vi "2P_AdapUprite_Linlin.vi"() -> ()   [LabVIEW 2015] (continued)
                                n912 = disable-structure shown="Disabled" {
                                frame Disabled {
                                n913 = call "stoperaseCI.vi"() -> ()  [unwired: 12 in]
                                n914 = call "stoperaseDO_img.vi"() -> ()  [unwired: 12 in]
                                n915 = call "stoperaseAO_img.vi"() -> ()  [unwired: 12 in]
                                n916 = call "stoperaseAI_img.vi"() -> ()  [unwired: 12 in]
                                }
                                frame Enabled {
                                }
                                }
                                }
                                frame #1 {
                                n917 = disable-structure shown="Disabled" {
                                frame Disabled {
                                n918 = local read "Acquisition time"() -> (w3439:i32)
                                n919 = call "collect_allLT_img.vi"() -> ("counts"=w3441:i32)  [unwired: 1 out]
                                n920 = local read "counts"() -> (w3442:i32)
                                n921 = Add(x=w3442, y=w3441) -> (x+y=w3440:i32)
                                "counts" <- w3440
                                n922 = Divide(x=w3440, y=w3439) -> (x/y=w3438:dbl)
                                n923 = Multiply(x=1000.0, y=w3438) -> (x*y=w3437:dbl)
                                n924 = local write "Avg Counts/s"(w3437) -> ()
                                }
                                frame Enabled {
                                }
                                }
                                }
                                frame #2 {
                                w3445 = u16 0 items=["Stream to disk", "Post process", "real time process"] ("Ring")
                                n925 = local read "T3R Data processing"() -> (w3444:u16)
                                n926 = local read "save\ndata"() -> (w3447:bool)
                                n927 = Equal?(x=w3444, y=w3445) -> (x = y?=w3443:bool)
                                n928 = Not(x=w3443) -> (.not. x?=w3448:bool)
                                n929 = And(x=w3447, y=w3448) -> (x .and. y?=w3446:bool)
                                n930 = case shown="True" w3446 {
                                tunnel: w3449 -> [_ w3451]
                                frame False {
                                }
                                frame True {
                                n931 = local read "filename prefix"() -> (w3452:string)
                                n932 = local read "data dir"() -> (w3457:path)
                                n933 = call "2pparameters.vi"("command"="get") -> ("params out"=w3472:T12)  [unwired: 1 in]
                                n934 = call "generatedatafilename.vi"("timestamp"=w3451, "filename prefix in"=w3452) -> ("full-filename"=w3450:string)
                                n935 = Unbundle By Name(w3472) -> ("srate"=w3470:sgl, "sAOxy"=w3469:i32, "Xpixels Img"=w3467:i32, "Ypixels Img"=w3465:i32)
                                n936 = Concatenate Strings(w3450, ".lvpt3img" ("string")) -> (w3455:string)
                                n937 = Build Path(base path=w3457, name or relative path=w3455) -> (appended path=w3454:path)
                                n938 = To Unsigned Long Integer(number=w3470) -> (unsigned 32bit integer=w3471:u32)
                                n939 = To Unsigned Long Integer(number=w3469) -> (unsigned 32bit integer=w3468:u32)
                                n940 = To Unsigned Long Integer(number=w3467) -> (unsigned 32bit integer=w3466:u32)
                                n941 = To Unsigned Long Integer(number=w3465) -> (unsigned 32bit integer=w3464:u32)
                                n942 = call "PH-temp-raw.vi"("command"="get") -> ("array out"=w3463:u32[])  [unwired: 1 in]
                                n943 = Build Array (concatenate)(w3471, w3468, w3466, w3464, w3463) -> (w3462:u32[])
                                n944 = Open/Create/Replace File(file path (use dialog)=w3454, operation (0:open)=T9."replace or create") -> (refnum out=w3461:refnum<file>, error out=w3460:errorcluster)  [unwired: 4 in, 1 out]
                                n945 = Write to Binary File(file (use dialog)=w3461, data=w3462, error in=w3460, 5:FALSE ("prepend array or string size? (T)")) -> (refnum out=w3458:refnum<file>, error out=w3459:errorcluster)  [unwired: 2 in, 1 out]
                                n946 = Close File(refnum=w3458, error in=w3459) -> ()  [unwired: 2 out]
                                }
                                }
                                n947 = call "stoperaseLT_img.vi"() -> ()  [unwired: 1 in]
                                }
                                frame #3 {
                                w3478 = u16 1 items=["Stream to disk", "Post process", "real time process"] ("Ring")
                                n948 = local read "T3R Data processing"() -> (w3477:u16)
                                n949 = Equal?(x=w3477, y=w3478) -> (x = y?=w3476:bool)
                                n950 = case shown="True" w3476 {
                                frame False {
                                }
                                frame True {
                                # "intensity"
                                # "lifetime"
                                # "intensity"
                                n951 = property on="img_CH1" class="IntGraph (strict)"() -> ("Value"=w3491:sgl[][])  [unwired: 2 in, 2 out]
                                n952 = Array Max & Min(array=w3491) -> (max value=w3492:sgl)  [unwired: 3 out]
                                n953 = local read "lineshift"() -> (w3479:i32)
                                n954 = local read "min phot"() -> (w3493:u32)
                                n955 = To Unsigned Long Integer(number=w3492) -> (unsigned 32bit integer=w3495:u32)
                                n956 = local read "counts"() -> (w3481:i32)
                                n957 = call "wrapcutlifetime.vi"("lineshift"=w3479) -> ("pt3img"=w3490:u16[][], "lifetimes"=w3488:sgl[][], "okay"=w3483:bool, "# of frames"=w3480:i32)
                                "frames recorded" <- w3480
                                n958 = Greater?(x=w3493, y=w3495) -> (0:w3494:bool)
                                n959 = Quotient & Remainder(x=w3481, y=w3480) -> (floor(x/y)=w3482:i32)  [unwired: 1 out]
                                n960 = Transpose 2D Array(2D array=w3490) -> (transposed array=w3484:u16[][])
                                n961 = Transpose 2D Array(2D array=w3488) -> (transposed array=w3489:sgl[][])
                                n962 = And(x=w3494, y=w3483) -> (x .and. y?=w3496:bool)
                                n963 = local write "img_CH2"(w3489) -> ()
                                n964 = local write "photons/frame"(w3482) -> ()
                                n965 = Array Max & Min(array=w3484) -> (max value=w3485:u16)  [unwired: 3 out]
                                n966 = To Single Precision Float(number=w3484) -> (single precision float=w3487:sgl[][])
                                n967 = case shown="True" w3496 {
                                tunnel: w3495 -> [_ w3500]
                                frame False {
                                }
                                frame True {
                                n968 = Quotient & Remainder(x=w3500, y=u32 2 ("min phot")) -> (floor(x/y)=w3499:u32)  [unwired: 1 out]
                                n969 = Max & Min(x=w3499, y=u32 5) -> (max(x,y)=w3498:u32)  [unwired: 1 out]
                                n970 = local write "min phot"(w3498) -> ()
                                }
                                }
                                n971 = To Double Precision Float(number=w3485) -> (double precision float=w3486:dbl)
                                n972 = local write "img_CH1"(w3487) -> ()
                                n973 = property on="img_CH1" class="IntGraph (strict)"("ZScale.Maximum"=w3486) -> ()  [unwired: 2 in, 2 out]
                                }
                                }
                                }
                                frame #4 {
                                w3504 = u16 1 items=["Stream to disk", "Post process", "real time process"] ("Ring")
                                n974 = local read "T3R Data processing"() -> (w3503:u16)
                                n975 = Equal?(x=w3503, y=w3504) -> (x = y?=w3502:bool)
                                n976 = case shown="False" w3502 {
                                frame False {
                                # "intensity"
                                n977 = local read "Current Average"() -> (w3509:sgl)
                                n978 = local read "image2list"() -> (w3505:u16)
                                n979 = local read "image1list"() -> (w3506:u16)
                                n980 = call "dattoimage.vi"("image2list"=w3505, "Current Average"=w3509, "image1list"=w3506) -> ("image 1 array out"=w3508:sgl[][])  [unwired: 1 out]
                                n981 = Transpose 2D Array(2D array=w3508) -> (transposed array=w3507:sgl[][])
                                n982 = local write "img_CH2"(w3507) -> ()
                                }
                                frame True {
                                }
                                }
                                }
                                }
                              }
                              frame Enabled {
                              }
                            }
                          }
                        }
                        n983 = local write "64bit disabled"(TRUE ("64bit disabled")) -> ()
                      }
                      frame #9 {
                        # "Reset the AO values after scanning to a known state (possibly source of delay after pressing stop)"
                        n984 = call "2pparameters.vi"("command"="get") -> ("params out"=w3514:T12)  [unwired: 1 in]
                        n985 = Unbundle By Name(w3514) -> ("auto OD"=w3513:bool, "autoshutter"=w3511:bool, "aAS"=w3510:u32[])
                        n986 = case shown="True" w3513 {
                          frame False {
                          }
                          frame True {
                            n987 = call "configuration_2P_Linlin.vi"("command"="get") -> ("config out"=w3517:T14)  [unwired: 2 in, 1 out]
                            n988 = call "2pparameters.vi"("command"="get") -> ("params out"=w3522:T12)  [unwired: 1 in]
                            n989 = Unbundle By Name(w3517) -> ("image OD"=w3519:u16)
                            n990 = Unbundle By Name(w3522) -> ("ODfilt"=w3520:u16)
                            n991 = call "filterwheelcontrol_nothorlabslib.vi"("Current OD filt"=w3519, "New ODfilt"=w3520) -> ()  [unwired: 1 in]
                          }
                        }
                        n992 = case shown="True" w3511 {
                          tunnel: w3510 -> [_ w3515]
                          frame False {
                          }
                          frame True {
                            n993 = call "shuttercontrol_multi.vi"("Autoshutter Chans"=w3515, "command"="close") -> ()  [unwired: 1 in, 1 out]
                          }
                        }
                        n994 = disable-structure shown="Disabled" {
                          frame Disabled {
                            # "<- possible source of delay"
                            n995 = call "reset AO_DO_v3.vi"() -> ()  [unwired: 12 in]
                          }
                          frame Disabled {
                            # "<- possible source of delay"
                            n996 = call "reset AO_DO_v3.vi"() -> ()  [unwired: 12 in]
                          }
                          frame Enabled {
                          }
                        }
                        n997 = flat-sequence {
                          frame #0 {
                            n998 = call "reset AO_DO_v3.vi"() -> ()  [unwired: 12 in]
                          }
                          frame #1 {
                            n999 = call "stoperaseCI.vi"() -> ()  [unwired: 12 in]
                            n1000 = call "stoperaseDO_img.vi"() -> ()  [unwired: 12 in]
                            n1001 = call "stoperaseAO_img.vi"() -> ()  [unwired: 12 in]
                            n1002 = call "stoperaseAI_img.vi"() -> ()  [unwired: 12 in]
                          }
                        }
                      }
                      frame #10 {
                        # "CI: counter input (for photon counting)"
                        # "If waveform determined scan... separates out scanning waveforms from 'waveform generation' waveforms"
                        n1003 = stacked-sequence {
                          tunnel: w3536 -> [w3539 _ _ _ _ _]
                          tunnel: w3535 -> [w3538 _ _ _ _ _]
                          tunnel: w3534 -> [w3537 _ _ _ _ _]
                          tunnel: w3533 -> [_ w3588 _ _ _ _]
                          tunnel: w3532 -> [_ w3587 w3642 w3759 _ _]
                          tunnel: w3531 -> [_ w3586 w3641 w3758 _ _]
                          tunnel: w3530 -> [_ _ w3640 _ _ _]
                          tunnel: w3529 -> [_ _ w3639 _ _ _]
                          tunnel: w3528 -> [_ _ _ w3757 _ _]
                          tunnel: w3527 -> [_ _ _ w3756 _ _]
                          tunnel: w3526 -> [_ _ w3637 _ _ _]
                          tunnel: w3525 -> [_ _ w3636 _ _ _]
                          tunnel: w3524 -> [_ _ _ w3754 _ _]
                          tunnel: w3523 -> [_ _ _ w3753 _ _]
                          frame #0 {
                            # "Whether X galvo was added"
                            n1004 = case shown="False" w3539 {
                              tunnel: w3538 -> [_ w3561]
                              tunnel: w3537 -> [_ w3560]
                              frame True {
                                # "If added, remove it from wf parameters and add it to wave forms AO"
                                n1005 = stacked-sequence {
                                seq-local: [w3542 _ _] -> [_ w3552 w3557]
                                frame #0 {
                                n1006 = call "configuration_2P_Linlin.vi"("command"="get") -> ("config out"=w3540:T14)  [unwired: 2 in, 1 out]
                                n1007 = Unbundle By Name(w3540) -> ("Voltage to Xgalvo"=w3545:i32)
                                n1008 = call "2pparameters.vi"("command"="get") -> ("params out"=w3546:T12)  [unwired: 1 in]
                                n1009 = in-place {
                                in-place-border: w3545 -> [w3551]
                                in-place-border: [w3548] -> w3542
                                n1010 = in-place-cluster #9(w3546) -> ("aAO"=w3550:u32[])
                                n1011 = call "remove channel from active arrayv2.vi"("line array in"=w3550, "line to remove"=w3551) -> ("line array out"=w3549:u32[], "index"=w3548:i32)  [unwired: 1 out]
                                n1012 = in-place-cluster #9("aAO"=w3549) -> (w3543:T12)
                                }
                                n1013 = call "2pparameters.vi"("Params in"=w3543, "command"="set") -> ()  [unwired: 1 out]
                                }
                                frame #1 {
                                n1014 = call "waveformparamsv2.vi"("command"="rem AO", "index"=w3552) -> ()  [unwired: 3 in, 3 out]
                                }
                                frame #2 {
                                n1015 = call "waveformsAObuffer.vi"("command"="get") -> ("AO wf out"=w3558:waveform(dbl)[])  [unwired: 1 in]
                                n1016 = Delete From Array(array=w3558, length=1, index=w3557) -> (array with subset deleted=w3554:waveform(dbl)[])  [unwired: 1 out]
                                n1017 = call "waveformsAObuffer.vi"("AO wf in"=w3554, "command"="set") -> ()  [unwired: 1 out]
                                }
                                }
                              }
                              frame False {
                                # "If false, get it from AO parameters"
                                n1018 = stacked-sequence {
                                seq-local: [w3564 _ _] -> [_ w3570 w3581]
                                tunnel: w3561 -> [_ w3569 _]
                                tunnel: w3560 -> [_ _ w3580]
                                frame #0 {
                                n1019 = call "configuration_2P_Linlin.vi"("command"="get") -> ("config out"=w3562:T14)  [unwired: 2 in, 1 out]
                                n1020 = Unbundle By Name(w3562) -> ("Voltage to Xgalvo"=w3565:i32)
                                n1021 = call "2pparameters.vi"("command"="get") -> ("params out"=w3568:T12)  [unwired: 1 in]
                                n1022 = Unbundle By Name(w3568) -> ("aAO"=w3566:u32[])
                                n1023 = Search 1D Array(1D array=w3566, element=w3565) -> (index of element=w3564:i32)  [unwired: 1 in]
                                }
                                frame #1 {
                                n1024 = call "waveformparamsv2.vi"("command"="get") -> ("Params out"=w3573:T17)  [unwired: 4 in, 2 out]
                                n1025 = in-place {
                                in-place-border: w3570 -> [w3577]
                                in-place-border: w3569 -> [w3576]
                                n1026 = in-place-cluster #10(w3573) -> ("AO parameters"=w3578:T18)
                                n1027 = in-place {
                                in-place-border: w3576 -> [w3579]
                                n1028 = in-place-array #11(w3578, w3577) -> ()  [unwired: 1 out]
                                n1029 = in-place-array #11(w3579) -> (w3575:T18)  [unwired: 1 out]
                                }
                                n1030 = in-place-cluster #10("AO parameters"=w3575) -> (w3571:T17)
                                }
                                n1031 = call "waveformparamsv2.vi"("command"="set", "Params in"=w3571) -> ()  [unwired: 3 in, 3 out]
                                }
                                frame #2 {
                                n1032 = call "waveformsAObuffer.vi"("command"="get") -> ("AO wf out"=w3584:waveform(dbl)[])  [unwired: 1 in]
                                n1033 = Replace Array Subset(array=w3584, new element=w3580, index=w3581) -> (w3582:waveform(dbl)[])
                                n1034 = call "waveformsAObuffer.vi"("AO wf in"=w3582, "command"="set") -> ()  [unwired: 1 out]
                                }
                                }
                              }
                            }
                          }
                          frame #1 {
                            # "same as last frame but for Y galvo waveform"
                            n1035 = case shown="False" w3588 {
                              tunnel: w3587 -> [_ w3610]
                              tunnel: w3586 -> [_ w3609]
                              frame True {
                                n1036 = stacked-sequence {
                                seq-local: [w3591 _ _] -> [_ w3601 w3606]
                                frame #0 {
                                n1037 = call "configuration_2P_Linlin.vi"("command"="get") -> ("config out"=w3589:T14)  [unwired: 2 in, 1 out]
                                n1038 = Unbundle By Name(w3589) -> ("Voltage to Ygalvo"=w3594:i32)
                                n1039 = call "2pparameters.vi"("command"="get") -> ("params out"=w3595:T12)  [unwired: 1 in]
                                n1040 = in-place {
                                in-place-border: w3594 -> [w3600]
                                in-place-border: [w3597] -> w3591
                                n1041 = in-place-cluster #12(w3595) -> ("aAO"=w3599:u32[])
                                n1042 = call "remove channel from active arrayv2.vi"("line array in"=w3599, "line to remove"=w3600) -> ("line array out"=w3598:u32[], "index"=w3597:i32)  [unwired: 1 out]
                                n1043 = in-place-cluster #12("aAO"=w3598) -> (w3592:T12)
                                }
                                n1044 = call "2pparameters.vi"("Params in"=w3592, "command"="set") -> ()  [unwired: 1 out]
                                }
                                frame #1 {
                                n1045 = call "waveformparamsv2.vi"("command"="rem AO", "index"=w3601) -> ()  [unwired: 3 in, 3 out]
                                }
                                frame #2 {
                                n1046 = call "waveformsAObuffer.vi"("command"="get") -> ("AO wf out"=w3607:waveform(dbl)[])  [unwired: 1 in]
                                n1047 = Delete From Array(array=w3607, length=1, index=w3606) -> (array with subset deleted=w3603:waveform(dbl)[])  [unwired: 1 out]
                                n1048 = call "waveformsAObuffer.vi"("AO wf in"=w3603, "command"="set") -> ()  [unwired: 1 out]
                                }
                                }
                              }
                              frame False {
                                n1049 = stacked-sequence {
                                seq-local: [w3613 _ _] -> [_ w3619 w3630]
                                tunnel: w3610 -> [_ w3618 _]
                                tunnel: w3609 -> [_ _ w3629]
                                frame #0 {
                                n1050 = call "configuration_2P_Linlin.vi"("command"="get") -> ("config out"=w3611:T14)  [unwired: 2 in, 1 out]
                                n1051 = Unbundle By Name(w3611) -> ("Voltage to Ygalvo"=w3614:i32)
                                n1052 = call "2pparameters.vi"("command"="get") -> ("params out"=w3617:T12)  [unwired: 1 in]
                                n1053 = Unbundle By Name(w3617) -> ("aAO"=w3615:u32[])
                                n1054 = Search 1D Array(1D array=w3615, element=w3614) -> (index of element=w3613:i32)  [unwired: 1 in]
                                }
                                frame #1 {
                                n1055 = call "waveformparamsv2.vi"("command"="get") -> ("Params out"=w3622:T17)  [unwired: 4 in, 2 out]
                                n1056 = in-place {
                                in-place-border: w3619 -> [w3626]
                                in-place-border: w3618 -> [w3625]
                                n1057 = in-place-cluster #13(w3622) -> ("AO parameters"=w3627:T18)
                                n1058 = in-place {
                                in-place-border: w3625 -> [w3628]
                                n1059 = in-place-array #14(w3627, w3626) -> ()  [unwired: 1 out]
                                n1060 = in-place-array #14(w3628) -> (w3624:T18)  [unwired: 1 out]
                                }
                                n1061 = in-place-cluster #13("AO parameters"=w3624) -> (w3620:T17)
                                }
                                n1062 = call "waveformparamsv2.vi"("command"="set", "Params in"=w3620) -> ()  [unwired: 3 in, 3 out]
                                }
                                frame #2 {
                                n1063 = call "waveformsAObuffer.vi"("command"="get") -> ("AO wf out"=w3633:waveform(dbl)[])  [unwired: 1 in]
                                n1064 = Replace Array Subset(array=w3633, new element=w3629, index=w3630) -> (w3631:waveform(dbl)[])
                                n1065 = call "waveformsAObuffer.vi"("AO wf in"=w3631, "command"="set") -> ()  [unwired: 1 out]
                                }
                                }
                              }
                            }
                          }
                          frame #2 {
                            # "correctly output the  waveforms affected by both (autoshutter) and (waveform determined)"
                            n1066 = Build Array(w3637, w3636) -> (w3635:bool[])
                            n1067 = Boolean Array To Number(Boolean array=w3635) -> (number=w3638:u32)
                            n1068 = case shown="2" w3638 {
                              tunnel: w3642 -> [_ _ w3700]
                              tunnel: w3641 -> [_ _ w3699]
                              tunnel: w3640 -> [_ w3672 w3697]
                              tunnel: w3639 -> [_ w3671 w3698]
                              frame 1, Default {
                                n1069 = stacked-sequence {
                                seq-local: [w3645 _ _] -> [_ w3657 w3662]
                                frame #0 {
                                # "Remove autoshutter channel from DO list in 2p parameters"
                                n1070 = call "2pparameters.vi"("command"="get") -> ("params out"=w3644:T12)  [unwired: 1 in]
                                n1071 = Unbundle By Name(w3644) -> ("aAS"=w3643:u32[])
                                n1072 = for {
                                tunnel: [w3651] -> w3645 mode=indexing
                                tunnel: w3643 -> [w3649] mode=indexing
                                shift-right: [w3652] -> w3646
                                shift-left: w3644 -> [w3650]
                                n1073 = in-place {
                                in-place-border: w3649 -> [w3656]
                                in-place-border: [w3653] -> w3651
                                n1074 = in-place-cluster #15(w3650) -> ("aDO"=w3655:u32[])
                                n1075 = call "remove channel from active arrayv2.vi"("line array in"=w3655, "line to remove"=w3656) -> ("line array out"=w3654:u32[], "index"=w3653:i32)  [unwired: 1 out]
                                n1076 = in-place-cluster #15("aDO"=w3654) -> (w3652:T12)
                                }
                                }
                                n1077 = call "2pparameters.vi"("Params in"=w3646, "command"="set") -> ()  [unwired: 1 out]
                                }
                                frame #1 {
                                n1078 = for {
                                tunnel: w3657 -> [w3658] mode=indexing
                                n1079 = call "waveformparamsv2.vi"("command"="rem DO", "index"=w3658) -> ()  [unwired: 3 in, 3 out]
                                }
                                }
                                frame #2 {
                                # "sort so it removes the last elements first\nand does not mess up the order"
                                # "Remove waveforms of autoshutter channels from wave forms DO"
                                n1080 = call "waveformsDObuffer.vi"("command"="get") -> ("DO wf out"=w3665:digitalwaveform[])  [unwired: 1 in]
                                n1081 = Sort 1D Array(array=w3662) -> (sorted array=w3661:i32[])
                                n1082 = Reverse 1D Array(array=w3661) -> (reversed array=w3660:i32[])
                                n1083 = for {
                                tunnel: w3660 -> [w3667] mode=indexing
                                shift-right: [w3668] -> w3663
                                shift-left: w3665 -> [w3670]
                                n1084 = Delete From Array(array=w3670, length=1, index=w3667) -> (array with subset deleted=w3668:digitalwaveform[])  [unwired: 1 out]
                                }
                                n1085 = call "waveformsDObuffer.vi"("DO wf in"=w3663, "command"="set") -> ()  [unwired: 1 out]
                                }
                                }
                              }
                              frame 2 {
                                n1086 = stacked-sequence {
                                tunnel: w3672 -> [_ w3684 _]
                                tunnel: w3671 -> [_ _ w3691]
                                frame #0 {
                                # "add autoshutter channels to digital out"
                                n1087 = call "2pparameters.vi"("command"="get") -> ("params out"=w3674:T12)  [unwired: 1 in]
                                n1088 = Unbundle By Name(w3674) -> ("aAS"=w3673:u32[])
                                n1089 = in-place {
                                in-place-border: w3673 -> [w3678]
                                n1090 = in-place-cluster #16(w3674) -> ("aDO"=w3680:u32[])
                                n1091 = for {
                                shift-right: [w3682] -> w3679
                                shift-left: w3680 -> [w3683]
                                tunnel: w3678 -> [w3681] mode=indexing
                                n1092 = call "add channel to active arrayv2.vi"("line array in"=w3683, "line to add"=w3681) -> ("line array out"=w3682:u32[])  [unwired: 2 out]
                                }
                                n1093 = in-place-cluster #16("aDO"=w3679) -> (w3675:T12)
                                }
                                n1094 = call "2pparameters.vi"("Params in"=w3675, "command"="set") -> ()  [unwired: 1 out]
                                }
                                frame #1 {
                                # "Not sure the correct way to add multiple sets of parameters..."
                                # "add autoshutter waveforms to wf parameters v2"
                                n1095 = disable-structure shown="Disabled" {
                                disable-tunnel: w3684 -> [w3686 _]
                                frame Disabled {
                                n1096 = for {
                                tunnel: w3686 -> [w3687] mode=indexing
                                n1097 = call "waveformparamsv2.vi"("command"="add DO", "add DO"=w3687) -> ()  [unwired: 3 in, 3 out]
                                }
                                }
                                frame Enabled {
                                }
                                }
                                n1098 = call "waveformparamsv2.vi"("command"="add DO", "add DO"=w3684) -> ()  [unwired: 3 in, 3 out]
                                }
                                frame #2 {
                                # "add autoshutter waveforms to wave forms DO"
                                n1099 = call "waveformsDObuffer.vi"("command"="get") -> ("DO wf out"=w3692:digitalwaveform[])  [unwired: 1 in]
                                n1100 = for {
                                tunnel: w3691 -> [w3695] mode=indexing
                                shift-right: [w3694] -> w3689
                                shift-left: w3692 -> [w3696]
                                n1101 = Build Array (concatenate)(w3696, w3695) -> (w3694:digitalwaveform[])
                                }
                                n1102 = call "waveformsDObuffer.vi"("DO wf in"=w3689, "command"="set") -> ()  [unwired: 1 out]
                                }
                                }
                              }
                              frame 0 {
                                n1103 = stacked-sequence {
                                seq-local: [w3702 _ _] -> [_ w3710 w3734]
                                tunnel: w3700 -> [_ _ _]
                                tunnel: w3699 -> [_ _ _]
                                tunnel: w3698 -> [_ _ w3733]
                                tunnel: w3697 -> [_ w3709 _]
                                frame #0 {
                                n1104 = call "2pparameters.vi"("command"="get") -> ("params out"=w3705:T12)  [unwired: 1 in]
                                n1105 = Unbundle By Name(w3705) -> ("aDO"=w3703:u32[], "aAS"=w3701:u32[])
                                n1106 = for {
                                tunnel: w3703 -> [w3708]
                                tunnel: [w3707] -> w3702 mode=indexing
                                tunnel: w3701 -> [w3706] mode=indexing
                                n1107 = Search 1D Array(1D array=w3708, element=w3706) -> (index of element=w3707:i32)  [unwired: 1 in]
                                }
                                }
                                frame #1 {
                                n1108 = call "2pparameters.vi"("command"="get") -> ("params out"=w3713:T12)  [unwired: 1 in]
                                n1109 = Unbundle By Name(w3713) -> ("wavdet"=w3711:bool, "autoshutter"=w3712:bool)
                                n1110 = case shown="True" w3712 {
                                tunnel: w3710 -> [_ w3717]
                                tunnel: w3711 -> [_ w3716]
                                tunnel: w3709 -> [_ w3715]
                                frame False {
                                }
                                frame True {
                                n1111 = case shown="False" w3716 {
                                tunnel: w3717 -> [w3719 _]
                                tunnel: w3715 -> [w3718 _]
                                frame False {
                                # "Replace autoshutter channel DO waveforms with those that were generated from autoshutter."
                                n1112 = call "waveformparamsv2.vi"("command"="get") -> ("Params out"=w3722:T17)  [unwired: 4 in, 2 out]
                                n1113 = in-place {
                                in-place-border: w3719 -> [w3726]
                                in-place-border: w3718 -> [w3724]
                                n1114 = in-place-cluster #17(w3722) -> ("DO parameters"=w3727:T20)
                                n1115 = for {
                                tunnel: w3726 -> [w3730] mode=indexing
                                tunnel: w3724 -> [w3728] mode=indexing
                                shift-right: [w3729] -> w3725
                                shift-left: w3727 -> [w3731]
                                n1116 = in-place {
                                in-place-border: w3728 -> [w3732]
                                n1117 = in-place-array #18(w3731, w3730) -> ()  [unwired: 1 out]
                                n1118 = in-place-array #18(w3732) -> (w3729:T20)  [unwired: 1 out]
                                }
                                }
                                n1119 = in-place-cluster #17("DO parameters"=w3725) -> (w3720:T17)
                                }
                                n1120 = call "waveformparamsv2.vi"("command"="set", "Params in"=w3720) -> ()  [unwired: 3 in, 3 out]
                                }
                                frame True {
                                }
                                }
                                }
                                }
                                }
                                frame #2 {
                                n1121 = call "2pparameters.vi"("command"="get") -> ("params out"=w3737:T12)  [unwired: 1 in]
                                n1122 = Unbundle By Name(w3737) -> ("wavdet"=w3735:bool, "autoshutter"=w3736:bool)
                                n1123 = case shown="True" w3736 {
                                tunnel: w3734 -> [_ w3741]
                                tunnel: w3735 -> [_ w3740]
                                tunnel: w3733 -> [_ w3739]
                                frame False {
                                }
                                frame True {
                                n1124 = case shown="False" w3740 {
                                tunnel: w3741 -> [w3743 _]
                                tunnel: w3739 -> [w3742 _]
                                frame False {
                                # "replace autoshutter channels of waveforms DO with autoshutter waveforms"
                                n1125 = call "waveformsDObuffer.vi"("command"="get") -> ("DO wf out"=w3745:digitalwaveform[])  [unwired: 1 in]
                                n1126 = for {
                                tunnel: w3743 -> [w3749] mode=indexing
                                tunnel: w3742 -> [w3748] mode=indexing
                                shift-right: [w3751] -> w3747
                                shift-left: w3745 -> [w3750]
                                n1127 = Replace Array Subset(array=w3750, new element=w3748, index=w3749) -> (w3751:digitalwaveform[])
                                }
                                n1128 = call "waveformsDObuffer.vi"("DO wf in"=w3747, "command"="set") -> ()  [unwired: 1 out]
                                }
                                frame True {
                                }
                                }
                                }
                                }
                                }
                                }
                              }
                            }
                          }
                          frame #3 {
                            # "Same thing for LT timestamp (?what is that?)"
                            n1129 = Build Array(w3754, w3753) -> (w3755:bool[])
                            n1130 = Boolean Array To Number(Boolean array=w3755) -> (number=w3752:u32)
                            n1131 = case shown="0" w3752 {
                              tunnel: w3759 -> [_ _ w3802]
                              tunnel: w3758 -> [_ _ w3801]
                              tunnel: w3757 -> [_ w3781 w3799]
                              tunnel: w3756 -> [_ w3780 w3800]
                              frame 1, Default {
                                n1132 = stacked-sequence {
                                seq-local: [w3762 _ _] -> [_ w3772 w3777]
                                frame #0 {
                                n1133 = call "configuration_2P_Linlin.vi"("command"="get") -> ("config out"=w3760:T14)  [unwired: 2 in, 1 out]
                                n1134 = Unbundle By Name(w3760) -> ("LT timestamp"=w3765:u32)
                                n1135 = call "2pparameters.vi"("command"="get") -> ("params out"=w3766:T12)  [unwired: 1 in]
                                n1136 = in-place {
                                in-place-border: w3765 -> [w3771]
                                in-place-border: [w3768] -> w3762
                                n1137 = in-place-cluster #19(w3766) -> ("aDO"=w3770:u32[])
                                n1138 = call "remove channel from active arrayv2.vi"("line array in"=w3770, "line to remove"=w3771) -> ("line array out"=w3769:u32[], "index"=w3768:i32)  [unwired: 1 out]
                                n1139 = in-place-cluster #19("aDO"=w3769) -> (w3763:T12)
                                }
                                n1140 = call "2pparameters.vi"("Params in"=w3763, "command"="set") -> ()  [unwired: 1 out]
                                }
                                frame #1 {
                                n1141 = call "waveformparamsv2.vi"("command"="rem DO", "index"=w3772) -> ()  [unwired: 3 in, 3 out]
                                }
                                frame #2 {
                                n1142 = call "waveformsDObuffer.vi"("command"="get") -> ("DO wf out"=w3778:digitalwaveform[])  [unwired: 1 in]
                                n1143 = Delete From Array(array=w3778, length=1, index=w3777) -> (array with subset deleted=w3774:digitalwaveform[])  [unwired: 1 out]
                                n1144 = call "waveformsDObuffer.vi"("DO wf in"=w3774, "command"="set") -> ()  [unwired: 1 out]
                                }
                                }
                              }
                              frame 2 {
                                n1145 = stacked-sequence {
                                tunnel: w3781 -> [_ _ w3794]
                                tunnel: w3780 -> [_ w3792 _]
                                frame #0 {
                                n1146 = call "configuration_2P_Linlin.vi"("command"="get") -> ("config out"=w3782:T14)  [unwired: 2 in, 1 out]
                                n1147 = Unbundle By Name(w3782) -> ("LT timestamp"=w3784:u32)
                                n1148 = call "2pparameters.vi"("command"="get") -> ("params out"=w3787:T12)  [unwired: 1 in]
                                n1149 = in-place {
                                in-place-border: w3784 -> [w3791]
                                n1150 = in-place-cluster #20(w3787) -> ("aDO"=w3790:u32[])
                                n1151 = call "add channel to active arrayv2.vi"("line array in"=w3790, "line to add"=w3791) -> ("line array out"=w3789:u32[])  [unwired: 2 out]
                                n1152 = in-place-cluster #20("aDO"=w3789) -> (w3785:T12)
                                }
                                n1153 = call "2pparameters.vi"("Params in"=w3785, "command"="set") -> ()  [unwired: 1 out]
                                }
                                frame #1 {
                                n1154 = call "waveformparamsv2.vi"("command"="add DO", "add DO"=w3792) -> ()  [unwired: 3 in, 3 out]
                                }
                                frame #2 {
                                n1155 = call "waveformsDObuffer.vi"("command"="get") -> ("DO wf out"=w3797:digitalwaveform[])  [unwired: 1 in]
                                n1156 = Build Array (concatenate)(w3797, w3794) -> (w3796:digitalwaveform[])
                                n1157 = call "waveformsDObuffer.vi"("DO wf in"=w3796, "command"="set") -> ()  [unwired: 1 out]
                                }
                                }
                              }
                              frame 0 {
                                n1158 = stacked-sequence {
                                seq-local: [w3805 _ _] -> [_ w3813 w3830]
                                tunnel: w3802 -> [_ _ _]
                                tunnel: w3801 -> [_ _ _]
                                tunnel: w3800 -> [_ w3810 _]
                                tunnel: w3799 -> [_ _ w3829]
                                frame #0 {
                                n1159 = call "configuration_2P_Linlin.vi"("command"="get") -> ("config out"=w3803:T14)  [unwired: 2 in, 1 out]
                                n1160 = Unbundle By Name(w3803) -> ("LT timestamp"=w3806:u32)
                                n1161 = call "2pparameters.vi"("command"="get") -> ("params out"=w3809:T12)  [unwired: 1 in]
                                n1162 = Unbundle By Name(w3809) -> ("aDO"=w3807:u32[])
                                n1163 = Search 1D Array(1D array=w3807, element=w3806) -> (index of element=w3805:i32)  [unwired: 1 in]
                                }
                                frame #1 {
                                n1164 = local read "Measurement"() -> (w3812:T4)
                                n1165 = To Unsigned Long Integer(number=w3812) -> (unsigned 32bit integer=w3811:u32)
                                n1166 = case shown="5..7" w3811 {
                                tunnel: w3813 -> [_ w3817]
                                tunnel: w3810 -> [_ w3814]
                                frame 0..4, Default {
                                }
                                frame 5..7 {
                                n1167 = Index Array(array=w3814, index=0) -> (element=w3815:T21)
                                n1168 = call "waveformparamsv2.vi"("command"="get") -> ("Params out"=w3820:T17)  [unwired: 4 in, 2 out]
                                n1169 = in-place {
                                in-place-border: w3817 -> [w3824]
                                in-place-border: w3815 -> [w3822]
                                n1170 = in-place-cluster #21(w3820) -> ("DO parameters"=w3825:T20)
                                n1171 = in-place {
                                in-place-border: w3822 -> [w3826]
                                n1172 = in-place-array #22(w3825, w3824) -> ()  [unwired: 1 out]
                                n1173 = in-place-array #22(w3826) -> (w3823:T20)  [unwired: 1 out]
                                }
                                n1174 = in-place-cluster #21("DO parameters"=w3823) -> (w3818:T17)
                                }
                                n1175 = call "waveformparamsv2.vi"("command"="set", "Params in"=w3818) -> ()  [unwired: 3 in, 3 out]
                                }
                                }
                                }
                                frame #2 {
                                n1176 = local read "Measurement"() -> (w3828:T4)
                                n1177 = To Unsigned Long Integer(number=w3828) -> (unsigned 32bit integer=w3827:u32)
                                n1178 = case shown="5..7" w3827 {
                                tunnel: w3830 -> [_ w3834]
                                tunnel: w3829 -> [_ w3832]
                                frame 0..4, Default {
                                }
                                frame 5..7 {
                                n1179 = Index Array(array=w3832, index=0) -> (element=w3831:digitalwaveform)
                                n1180 = call "waveformsDObuffer.vi"("command"="get") -> ("DO wf out"=w3836:digitalwaveform[])  [unwired: 1 in]
                                n1181 = Replace Array Subset(array=w3836, new element=w3831, index=w3834) -> (w3838:digitalwaveform[])
                                n1182 = call "waveformsDObuffer.vi"("DO wf in"=w3838, "command"="set") -> ()  [unwired: 1 out]
                                }
                                }
                                }
                                }
                              }
                            }
                          }
                          frame #4 {
                            # "Looks like its updating the waveforms pallette with relevant info"
                            n1183 = call "Used AO lines.vi"() -> ("used AO names"=w3841:string[], "used AO lines"=w3839:tag[])  [unwired: 2 in]
                            n1184 = control-ref of="Analog Lines Plot"() -> (w3840:refnum<vi>)
                            n1185 = control-ref of="Digital Lines Plot"() -> (w3842:refnum<vi>)
                            n1186 = call "Used DO lines.vi"() -> ("used DO names"=w3843:string[], "used DO lines"=w3844:tag[])  [unwired: 2 in]
                            n1187 = local write "Analog Used Lines"(w3839) -> ()
                            n1188 = local write "Analog Used Names"(w3841) -> ()
                            n1189 = local write "Digital Used Lines"(w3844) -> ()
                            n1190 = local write "Digital Used Names"(w3843) -> ()
                            n1191 = call "prepDOWaveplot.vi"("DigitalGraph in"=w3842, "used DO names"=w3843) -> ()  [unwired: 1 in]
                            n1192 = call "prepAOWaveplot.vi"("WaveformGraph in"=w3840, "Analog Used Names"=w3841) -> ()  [unwired: 1 in]
                          }
                          frame #5 {
                            # "Could this be source of crashing?"
                            n1193 = local read "Meastab"() -> (w3859:enum32{"X-Y Image", "Linescan", "Timetrace"})
                            n1194 = property on="refwf" class="Ring (strict)"() -> ("RingText.Text"=w3856:string)  [unwired: 2 in, 2 out]
                            n1195 = case shown="\"Timetrace\"" w3859 {
                              tunnel: [w3861 w3862] -> w3860
                              frame "X-Y Image", Default {
                                n1196 = local read "Sampling rate"() -> (w3861:dbl)
                              }
                              frame "Timetrace" {
                                n1197 = local read "srateAODOtt"() -> (w3862:dbl)
                              }
                            }
                            n1198 = call "waveformsAObuffer.vi"("command"="get") -> ("AO wf out"=w3847:waveform(dbl)[])  [unwired: 1 in]
                            n1199 = local read "wavdet"() -> (w3857:bool)
                            n1200 = call "waveformsDObuffer.vi"("command"="get") -> ("DO wf out"=w3851:digitalwaveform[])  [unwired: 1 in]
                            n1201 = call "correctwaveformsizetemp.vi"("new sampling frequency (Hz)"=w3860, "start"=FALSE, "reference waveforms to"=w3856, "Analog waveforms in"=w3847, "stop"=TRUE, "Digital waveforms in"=w3851) -> ("analog wf out"=w3853:waveform(dbl)[], "Digital wf out"=w3855:digitalwaveform[], "measpoints"=w3858:i32)
                            n1202 = local write "Analog Lines Plot"(w3853) -> ()
                            n1203 = call "GetNumCamFramesv2.vi"("Digital Waveform Graph"=w3855) -> ("Numeric"=w3854:i32)  [unwired: 10 in]
                            n1204 = local write "Digital Lines Plot"(w3855) -> ()
                            n1205 = call "waveformsDObuffer.vi"("DO wf in"=w3855, "command"="set") -> ()  [unwired: 1 out]
                            n1206 = call "waveformsAObuffer.vi"("AO wf in"=w3853, "command"="set") -> ()  [unwired: 1 out]
                            n1207 = local write "Total Camera Frames"(w3854) -> ()
                            n1208 = case shown="True" w3857 {
                              tunnel: w3858 -> [_ w3863]
                              frame False {
                              }
                              frame True {
                                n1209 = local write "# of frames"(w3863) -> ()
                              }
                            }
                          }
                        }
                      }
                      frame #11 {
                        w3871 = FALSE ("Value (Signaling)")
                        # "Cleanup... saves parameters and timestamps to a file and closes the file to which TIFFs are saved"
                        n1210 = local read "save\ndata"() -> (w3864:bool)
                        n1211 = local read "save\ndata"() -> (w3865:bool)
                        n1212 = property on="Stop" class="Bool (strict)"("Visible"=FALSE, "DisabledEnum"=T7."Disabled" ("Disabled")) -> ()  [unwired: 2 in, 2 out]
                        n1213 = case shown="True" w3864 {
                          frame False {
                          }
                          frame True {
                            n1214 = call "closetiffs.vi"() -> ()  [unwired: 12 in]
                          }
                        }
                        n1215 = case shown="True" w3865 {
                          tunnel: w3866 -> [_ w3874]
                          frame False {
                          }
                          frame True {
                            n1216 = local read "filename prefix"() -> (w3872:string)
                            n1217 = local read "data dir"() -> (w3873:path)
                            n1218 = call "savetimestamps.vi"("timestamp"=w3874, "filename prefix in"=w3872, "data dir in"=w3873) -> ()  [unwired: 1 in]
                            n1219 = call "saveparams_andscanpattern.vi"("filename prefix in"=w3872, "data dir in"=w3873) -> ()  [unwired: 2 in]
                            n1220 = disable-structure shown="Disabled" {
                              disable-tunnel: w3873 -> [w3876 _]
                              disable-tunnel: w3872 -> [w3875 _]
                              frame Disabled {
                                n1221 = call "saveparams.vi"("filename prefix in"=w3875, "data dir in"=w3876) -> ()  [unwired: 2 in]
                              }
                              frame Enabled {
                              }
                            }
                          }
                        }
                        n1222 = property on="Start" class="Bool (strict)"("Visible"=TRUE, "DisabledEnum"=T7."Enabled" ("Disabled")) -> ()  [unwired: 2 in, 2 out]
                        n1223 = property on="Start" class="Bool (strict)"("Val(Sgnl)"=w3871) -> ()  [unwired: 2 in, 2 out]
                        n1224 = property on="Stop" class="Bool (strict)"("Val(Sgnl)"=w3871) -> ()  [unwired: 2 in, 2 out]
                      }
                      frame #12 {
                        w3880 = T24 2 items=["no dialog", "OK message", "continue or stop message", "OK message + warnings", "continue/stop + warnings"] ("type of dialog (OK msg:1)")
                        # "Error handling"
                        n1225 = call "displayerrors.vi"() -> ("error IO"=w3879:errorcluster)
                        n1226 = call <vilib>:"General Error Handler.vi"("type of dialog (OK msg:1)"=w3880, "error in (no error)"=w3879) -> ("error out"=w3878:errorcluster)  [unwired: 9 in, 4 out]
                        n1227 = call <vilib>:"Clear Errors.vi"("error in (no error)"=w3878) -> ("error out"=w3877:errorcluster)  [unwired: 5 in, 1 out]
                        n1228 = call "seterrors.vi"("error IO"=w3877) -> ()
                      }
                    }
                  }
                  frame "X-Y-Z-t movie" {
                    n1229 = call "2pparameters.vi"("command"="get") -> ("params out"=w3883:T12)  [unwired: 1 in]
                    n1230 = Bundle By Name(cluster=w3883, "type"="X-Y-Z-t movie") -> (w3881:T12)
                    n1231 = call "2pparameters.vi"("Params in"=w3881, "command"="set") -> ()  [unwired: 1 out]
                  }
                  frame "linescan" {
                    n1232 = call "2pparameters.vi"("command"="get") -> ("params out"=w3888:T12)  [unwired: 1 in]
                    n1233 = Bundle By Name(cluster=w3888, "type"="linescan") -> (w3890:T12)
                    n1234 = call "2pparameters.vi"("Params in"=w3890, "command"="set") -> ()  [unwired: 1 out]
                  }
                  frame "Timetrace", "Lifetime (contour)" {
                    n1235 = local read "ttt"() -> (w3891:T3)
                    n1236 = case shown="\"Point\", \"Resonant Ellipse\", \"freeform contour\", \"Fill Ellipse\", Default" w3891 {
                      selector: w3891 -> [_ w3892]
                      frame "Line" {
                      }
                      frame "Point", "Resonant Ellipse", "freeform contour", "Fill Ellipse", Default {
                        n1237 = stacked-sequence {
                          seq-local: [w3908 _ _ _ _ _ _ _ _ _ _] -> [_ _ w4848 _ _ w4863 w4930 _ _ w5310 _]
                          seq-local: [w3907 _ _ _ _ _ _ _ _ _ _] -> [_ _ _ _ _ _ _ _ w4977 _ _]
                          seq-local: [w3906 _ _ _ _ _ _ _ _ _ _] -> [_ _ _ _ _ _ _ _ w4976 _ _]
                          seq-local: [w3905 _ _ _ _ _ _ _ _ _ _] -> [_ _ _ _ _ _ _ _ w4979 _ _]
                          seq-local: [w3904 _ _ _ _ _ _ _ _ _ _] -> [_ _ _ _ _ _ _ _ w4975 _ _]
                          seq-local: [w3903 _ _ _ _ _ _ _ _ _ _] -> [_ _ _ _ _ _ _ _ w4974 _ _]
                          seq-local: [w3902 _ _ _ _ _ _ _ _ _ _] -> [_ _ _ _ _ _ _ _ w4978 _ _]
                          seq-local: [w3901 _ _ _ _ _ _ _ _ _ _] -> [_ _ _ _ _ _ _ _ w4973 _ _]
                          seq-local: [w3900 _ _ _ _ _ _ _ _ _ _] -> [_ _ _ _ _ _ _ _ w4972 _ _]
                          seq-local: [w3899 _ _ _ _ _ _ _ _ _ _] -> [_ _ _ _ _ _ _ _ w4967 _ _]
                          seq-local: [w3898 _ _ _ _ _ _ _ _ _ _] -> [_ _ _ _ _ _ _ _ w4966 _ _]
                          seq-local: [w3897 _ _ _ _ _ _ _ _ _ _] -> [_ _ _ _ _ _ _ _ w4971 _ _]
                          seq-local: [w3896 _ _ _ _ _ _ _ _ _ _] -> [_ _ _ _ _ _ _ _ w4970 _ _]
                          seq-local: [w3895 _ _ _ _ _ _ _ _ _ _] -> [_ _ _ _ _ _ _ _ w4969 _ _]
                          seq-local: [w3894 _ _ _ _ _ _ _ _ _ _] -> [_ _ _ _ _ _ _ _ w4968 _ _]
                          tunnel: w3892 -> [w3893 _ _ _ _ _ _ _ _ _ _]
                          frame #0 {
                            n1238 = Get Date/Time In Seconds() -> (seconds since 1Jan1904=w3910:timestamp)
                            n1239 = local read "save\ndata"() -> (w3909:bool)
                            n1240 = case shown="False" w3909 {
                              tunnel: w3910 -> [w3911 w3913]
                              tunnel: [w3911 w3912] -> w3908
                              frame False {
                              }
                              frame True {
                                n1241 = call "createdatafolder.vi"("timestamp in"=w3913) -> ("current data path"=w3914:path, "timestamp out"=w3912:timestamp)
                                n1242 = local write "data dir"(w3914) -> ()
                              }
                            }
                            n1243 = stacked-sequence {
                              tunnel: w3908 -> [w3921 _ _ _ _ _ _ _ _]
                              tunnel: [_ _ _ _ _ _ w4121 _ _] -> w3907
                              tunnel: [_ _ _ _ _ _ w4120 _ _] -> w3906
                              tunnel: [_ _ _ _ _ _ w4119 _ _] -> w3905
                              tunnel: [_ _ _ _ _ _ w4118 _ _] -> w3904
                              tunnel: [_ _ _ _ _ _ w4117 _ _] -> w3903
                              tunnel: [_ _ _ _ _ _ w4116 _ _] -> w3902
                              tunnel: [_ _ _ _ _ _ w4115 _ _] -> w3901
                              tunnel: [_ _ _ _ _ _ w4114 _ _] -> w3900
                              tunnel: [_ _ _ _ _ _ w4113 _ _] -> w3899
                              tunnel: [_ _ _ _ _ _ w4112 _ _] -> w3898
                              tunnel: [_ _ _ _ _ _ w4111 _ _] -> w3897
                              tunnel: [_ _ _ _ _ _ w4110 _ _] -> w3896
                              tunnel: [_ _ _ _ _ _ w4109 _ _] -> w3895
                              tunnel: [_ _ _ _ _ _ w4108 _ _] -> w3894
                              tunnel: w3893 -> [_ _ w3960 _ w4012 _ _ _ _]
                              frame #0 {
                                # "creates date and time string... housekeeping"
                                n1244 = local read "Auto Shutter Channels"() -> (w3915:i32[])
                                n1245 = Format Date/Time String(time format string (%c)="%Y%m%d", seconds (now)=w3921) -> (date/time string=w3920:string)  [unwired: 1 in]
                                n1246 = Format Date/Time String(time format string (%c)="%H%M%S", seconds (now)=w3921) -> (date/time string=w3919:string)  [unwired: 1 in]
                                n1247 = local write "graphtab"(T8."timetrace" ("graphtab")) -> ()
                                n1248 = local read "AI channels"() -> (w3925:i32[])
                                n1249 = local read "CI channels"() -> (w3926:i32[])
                                n1250 = property on="Stop" class="Bool (strict)"("Visible"=TRUE, "DisabledEnum"=T7."Enabled" ("Disabled")) -> ()  [unwired: 2 in, 2 out]
                                n1251 = property on="Start" class="Bool (strict)"("Visible"=FALSE, "DisabledEnum"=T7."Disabled and Grayed Out" ("Disabled")) -> ()  [unwired: 2 in, 2 out]
                                n1252 = call "2pparameters.vi"("command"="get") -> ("params out"=w3928:T12)  [unwired: 1 in]
                                n1253 = Bundle By Name(cluster=w3928, "aAI"=w3925, "aCI"=w3926, "type"="Timetrace", "date"=w3920, "time"=w3919, "aAS"=w3915) -> (w3927:T12)
                                n1254 = call "X-array-databuffer.vi"("command"=enum16{"get", "set", "clear", "append"}."clear") -> ()  [unwired: 3 in, 2 out]
                                n1255 = call "Y-array-databuffer.vi"("command"=enum16{"get", "set", "clear", "append"}."clear") -> ()  [unwired: 3 in, 2 out]
                                n1256 = call "2pparameters.vi"("Params in"=w3927, "command"="set") -> ()  [unwired: 1 out]
                                n1257 = call "CH1-1D-temp.vi"("command"=enum16{"get", "set", "clear", "append"}."clear") -> ()  [unwired: 3 in, 2 out]
                                n1258 = call "CH2-1D-temp.vi"("command"=enum16{"get", "set", "clear", "append"}."clear") -> ()  [unwired: 3 in, 2 out]
                                n1259 = call "allAI-temp.vi"("command"=enum16{"get", "set", "clear", "append"}."clear") -> ()  [unwired: 3 in, 2 out]
                              }
                              frame #1 {
                                # "graph list for type of data to aquire"
                                n1260 = call "configuration_2P_Linlin.vi"("command"="get") -> ("config out"=w3938:T14)  [unwired: 2 in, 1 out]
                                n1261 = Unbundle By Name(w3938) -> ("CI names"=w3946:string[], "AI names"=w3947:string[])
                                n1262 = call "2pparameters.vi"("command"="get") -> ("params out"=w3943:T12)  [unwired: 1 in]
                                n1263 = Unbundle By Name(w3943) -> ("aCI"=w3944:i32[], "aAI"=w3945:i32[])
                                n1264 = for {
                                tunnel: w3944 -> [w3957] mode=indexing
                                tunnel: w3946 -> [w3958]
                                tunnel: [w3956] -> w3948 mode=indexing
                                n1265 = Index Array(array=w3958, index=w3957) -> (element=w3956:string)
                                }
                                n1266 = for {
                                tunnel: w3945 -> [w3954] mode=indexing
                                tunnel: w3947 -> [w3955]
                                tunnel: [w3953] -> w3949 mode=indexing
                                n1267 = Index Array(array=w3955, index=w3954) -> (element=w3953:string)
                                }
                                n1268 = Build Array (concatenate)(w3948, w3949) -> (w3941:string[])
                                n1269 = for {
                                tunnel: w3941 -> [w3951] mode=indexing
                                tunnel: [w3950] -> w3940 mode=indexing
                                i -> [w3952]
                                n1270 = Bundle("String"=w3951, w3952) -> (w3950:cluster{"String":string, i32})  [unwired: 1 in]
                                }
                                n1271 = property on="graph1list" class="Ring (strict)"("StringsAndValues[]"=w3940) -> ()  [unwired: 2 in, 2 out]
                                n1272 = property on="graph2list" class="Ring (strict)"("StringsAndValues[]"=w3940) -> ()  [unwired: 2 in, 2 out]
                              }
                              frame #2 {
                                # "OD wheel... doesnt work in 64bit labview"
                                n1273 = call "2pparameters.vi"("command"="get") -> ("params out"=w3963:T12)  [unwired: 1 in]
                                n1274 = Unbundle By Name(w3963) -> ("auto OD"=w3961:bool, "autoshutter"=w3964:bool, "aAS"=w3959:u32[])
                                n1275 = case shown="True" w3961 {
                                tunnel: w3960 -> [_ w3965]
                                frame False {
                                }
                                frame True {
                                n1276 = case shown="\"Point\"" w3965 {
                                frame "Point" {
                                }
                                frame "Resonant Ellipse", Default {
                                }
                                }
                                }
                                }
                                n1277 = case shown="True" w3964 {
                                tunnel: w3959 -> [_ w3966]
                                frame False {
                                }
                                frame True {
                                n1278 = call "shuttercontrol_multi.vi"("Autoshutter Chans"=w3966, "command"="close") -> ()  [unwired: 1 in, 1 out]
                                }
                                }
                              }
                              frame #3 {
                                # "takes all the relevant variables from the front page and puts them in a buffer structure"
                                n1279 = local read "Vy-min draw"() -> (w3975:dbl)
                                n1280 = local read "Vy-max draw"() -> (w3974:dbl)
                                n1281 = local read "Vx-min draw"() -> (w3977:dbl)
                                n1282 = local read "Vx-max draw"() -> (w3976:dbl)
                                n1283 = local read "xpixels ref"() -> (w3973:i32)
                                n1284 = local read "ypixels ref"() -> (w3972:i32)
                                n1285 = local read "ROI Type"() -> (w3971:u16)
                                n1286 = local read "srateAODOtt"() -> (w3994:dbl)
                                n1287 = local read "# of frames"() -> (w3999:i32)
                                n1288 = local read "refreshtime"() -> (w3991:dbl)
                                n1289 = local read "Pel"() -> (w3970:dbl)
                                n1290 = local read "bin"() -> (w3997:dbl)
                                n1291 = local read "Override AI buffer"() -> (w3968:bool)
                                n1292 = local read "finite samples"() -> (w4006:bool)
                                n1293 = local read "srateAODOtt"() -> (w3993:dbl)
                                n1294 = local read "srateAODOtt"() -> (w4000:dbl)
                                n1295 = local read "continuous"() -> (w4005:bool)
                                n1296 = local read "Angle ref"() -> (w3978:dbl)
                                n1297 = local read "wavdet"() -> (w4007:bool)
                                n1298 = local read "Vx-ref"() -> (w4002:dbl)
                                n1299 = local read "Vy-ref"() -> (w4004:dbl)
